vi "Notify PV Monitoring.vi"(8 "error in (no error)":errorcluster, 11 "CS++DIMMonitor in":refnum<class "CS++DIMMonitor.lvclass">) -> (0 "error out":errorcluster, 3 "CS++DIMMonitor out":refnum<class "CS++DIMMonitor.lvclass">)   [LabVIEW 2016, in "CS++DIMMonitor.lvlib" / "CS++DIMMonitor.lvclass"]
doc: "Notify PV monitoring readout."
uses:
  CS++DIMMonitor.lvclass
  C:/User/Brand/LVP/CSPP-Dev/Packages/CSPP_Core/Actors/CS++PVMonitor/CS++PVMonitor.lvclass
  CSPP_Core/Actors/CS++PVMonitor/CS++PVMonitor.lvclass/CS++PVMonitor.ctl
  CS++DIMMonitor.lvclass/CS++DIMMonitor.ctl
  <vilib>/ActorFramework/Message Enqueuer/Message Enqueuer.lvclass
  CSPP_Core/Actors/CS++PVMonitor Messages/CS++PVUpdate Msg/CS++PVUpdate Msg.lvclass
  CSPP_Core/Actors/CS++PVMonitor/CS++PVMonitor.lvclass
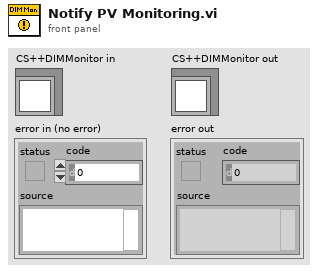
[diagram p1: front panel]
types:
  T1 = cluster{"PV URL":string, "Observers":cluster{"Enqueuer":refnum<class "Message Enqueuer.lvclass">, "CS++PVUpdate Msg":refnum<class "CS++PVUpdate Msg.lvclass">}[]}[]
  T2 = cluster{"DIM IDs":i32[], "PV Connections":cluster{"PV URL":string, "Observers":cluster{"Enqueuer":refnum<class "Message Enqueuer.lvclass">, "CS++PVUpdate Msg":refnum<class "CS++PVUpdate Msg.lvclass">}[]}[]}
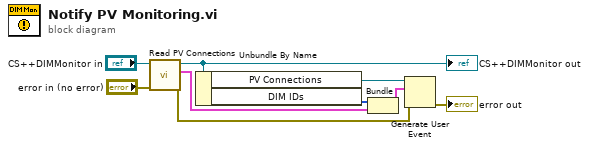
[diagram p0: block diagram]
diagram:
  n1 = call "Read PV Connections.vi"("error in (no error)"="error in (no error)", "CS++PVMonitor in"="CS++DIMMonitor in") -> ("error out"=w8:errorcluster, "PV Connections"=w6:T1, "CS++PVMonitor out"=w2:refnum<class "CS++DIMMonitor.lvclass">)  [unwired: 7 in]
  "CS++DIMMonitor out" <- w2
  n2 = Unbundle By Name(w2) -> ("PV Connections"=w7:refnum<user-event>, "DIM IDs"=w5:i32[])
  n3 = Bundle("DIM IDs"=w5, "PV Connections"=w6) -> (w9:T2)  [unwired: 1 in]
  n4 = Generate User Event(user event=w7, event data cluster=w9, error in=w8) -> (error out=→"error out":errorcluster)  [unwired: 1 in, 1 out]
